vi "Handle Command.vi"(8 "error in (no error)":errorcluster, 9 "Data":variant, 10 "Command":string, 11 "Inst.SPC in":refnum<class "Inst.SPC.lvclass">) -> (0 "error out":errorcluster, 1 "Processed Data":variant, 2 "Command":string, 3 "Inst.SPC out":refnum<class "Inst.SPC.lvclass">)   [LabVIEW 2019, in "Inst.SPC.lvclass"]
uses:
  Inst.SPC.lvclass
  9aec49fd-fe04-463a-be35-b7075f22e824.vi
  <userlib>/LevyLab/Instrument Framework/Instrument Types/VSource/Instrument.VSource.lvclass
  Typedefs/Inst.SPC.Configuration--Cluster.ctl
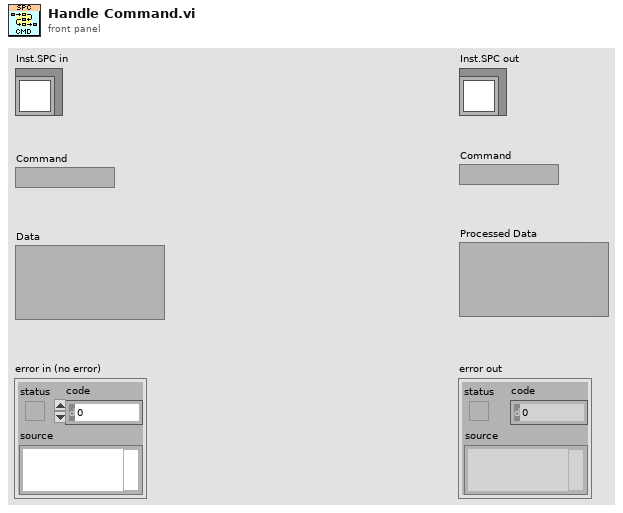
[diagram p1: front panel]
types:
  T1 = typedef "Inst.SPC.lvclass/Inst.SPC.Configuration--Cluster.ctl" = cluster{"DCC_DLL":path, "SPC_DLL":path, "DCC_Serials":string[], "SPC_Serials":string[]}
  T2 = typedef "Inst.SPC.lvclass/Inst.SPC.getAll--Cluster.ctl" = cluster{"DummyData":string}
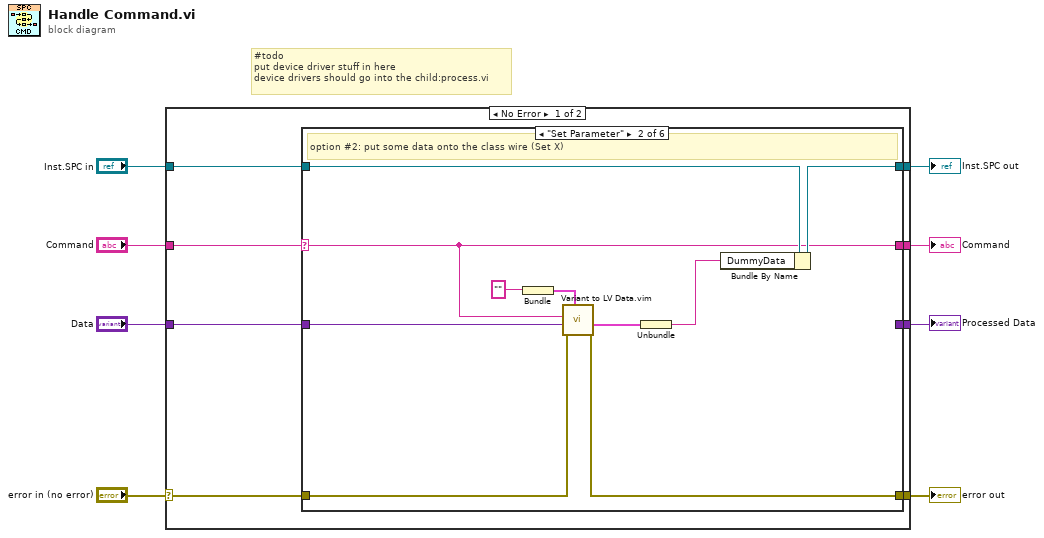
[diagram p0: block diagram]
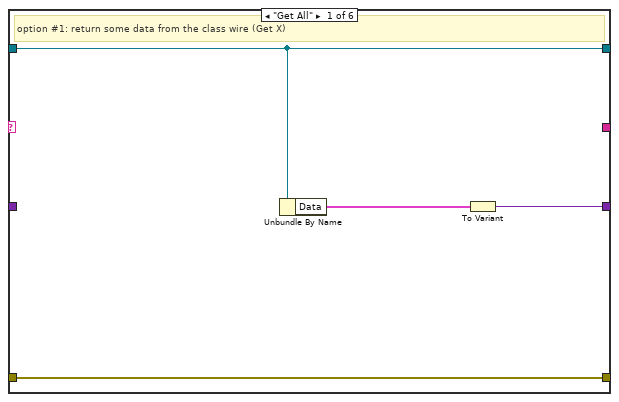
[diagram p2: hidden frame]
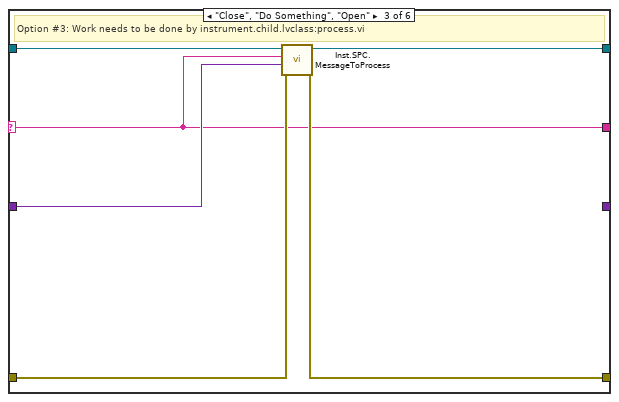
[diagram p3: hidden frame]
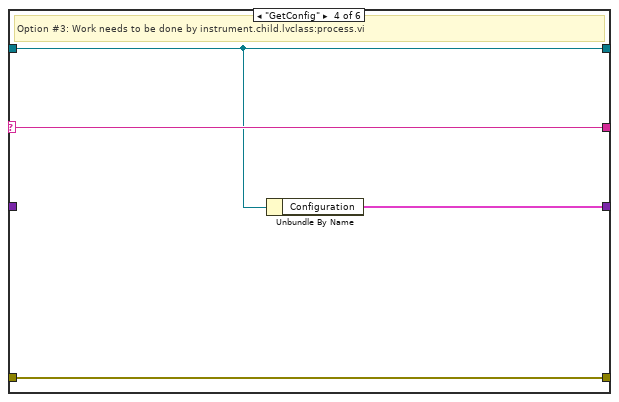
[diagram p4: hidden frame]
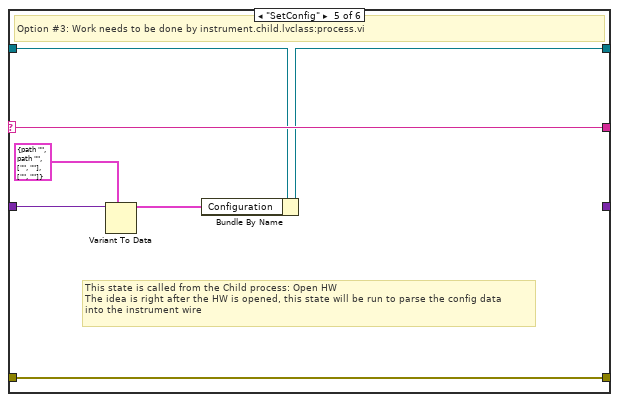
[diagram p5: hidden frame]
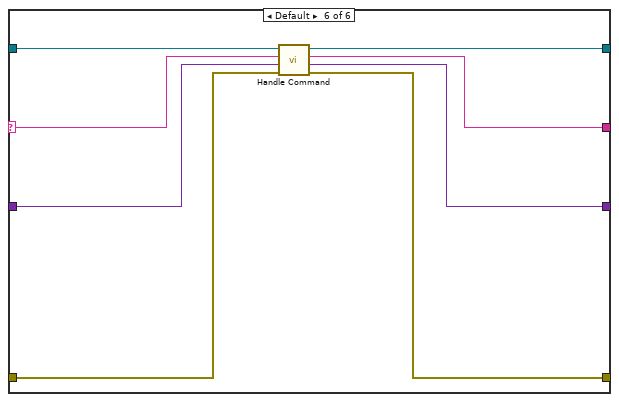
[diagram p6: hidden frame]
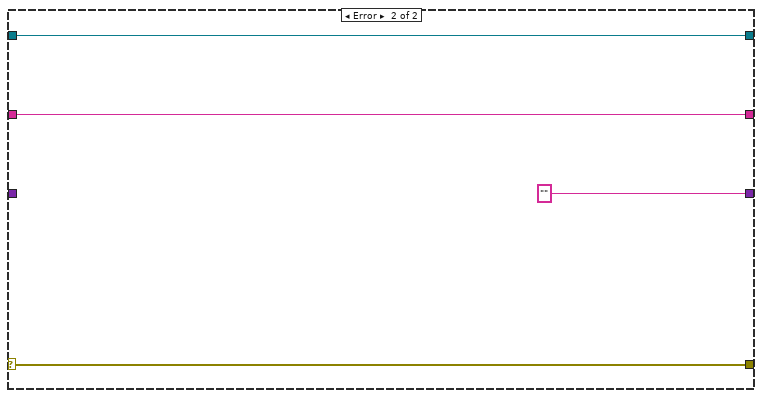
[diagram p7: hidden frame]
diagram:
  # "#todo\nput device driver stuff in here\ndevice drivers should go into the child:process.vi"
  n1 = case shown="No Error" "error in (no error)" {
    selector: "error in (no error)" -> [w10 w59]
    tunnel: [w12 w59] -> w6
    tunnel: [w14 w58] -> w5
    tunnel: "Inst.SPC in" -> [w15 w58]
    tunnel: "Command" -> [w16 w56]
    tunnel: [w13 "" ("String")] -> w3
    tunnel: "Data" -> [w9 _]
    tunnel: [w11 w56] -> w1
    frame No Error {
      n2 = case shown="\"Set Parameter\"" w16 {
        selector: w16 -> [_ w25 w31 w40 w47 w49]
        tunnel: w15 -> [w19 w30 w36 w38 w45 w53]
        tunnel: [w19 w29 w35 w38 w44 w50] -> w14
        tunnel: [w17 _ _ w39 _ w52] -> w13
        tunnel: w10 -> [w18 w28 w34 w37 w46 w54]
        tunnel: w9 -> [_ w26 w32 _ w43 w55]
        tunnel: [w18 w27 w33 w37 w46 w51] -> w12
        tunnel: [_ w25 w31 w40 w47 w48] -> w11
        frame "Get All" {
          # "option #1: return some data from the class wire (Get X)"
          n3 = Unbundle By Name(w19) -> ("Data"=w20:T2)
          n4 = To Variant(anything=w20) -> (Variant=w17:variant)
        }
        frame "Set Parameter" {
          # "option #2: put some data onto the class wire (Set X)"
          n5 = Bundle("") -> (w23:cluster{string})  [unwired: 1 in]
          n6 = call "Variant to LV Data.vim"("type"=w23, "error in (no error)"=w28, "JSON Data in"=w26, "Command"=w25) -> ("error out"=w27:errorcluster, "Data out"=w22:cluster{string})  [unwired: 4 in, 2 out]
          n7 = Unbundle(w22) -> (w21:string)
          n8 = Bundle By Name(cluster=w30, "DummyData"=w21) -> (w29:refnum<class "Inst.SPC.lvclass">)
        }
        frame "Close", "Do Something", "Open" {
          # "Option #3: Work needs to be done by instrument.child.lvclass:process.vi"
          n9 = call "Inst.SPC.MessageToProcess.vi"("error in (no error)"=w34, "Data"=w32, "Command"=w31, "Inst.SPC in"=w36) -> ("error out"=w33:errorcluster, "Inst.SPC out"=w35:refnum<class "Inst.SPC.lvclass">)  [unwired: 6 in]
        }
        frame "GetConfig" {
          # "Option #3: Work needs to be done by instrument.child.lvclass:process.vi"
          n10 = Unbundle By Name(w38) -> ("Configuration"=w39:T1)
        }
        frame "SetConfig" {
          # "This state is called from the Child process: Open HW\nThe idea is right after the HW is opened, this state will be run to parse the config data \ninto the instrument wire"
          # "Option #3: Work needs to be done by instrument.child.lvclass:process.vi"
          n11 = Variant To Data(type=T1 {"DCC_DLL"=path "", "SPC_DLL"=path "", "DCC_Serials"=["", ""], "SPC_Serials"=["", ""]} ("Configuration"), Variant=w43) -> (data=w42:T1)  [unwired: 1 in, 1 out]
          n12 = Bundle By Name(cluster=w45, "Configuration"=w42) -> (w44:refnum<class "Inst.SPC.lvclass">)
        }
        frame Default {
          n13 = call-parent "Handle Command.vi"("error in (no error)"=w54, "Data"=w55, "Command"=w49, "Instrument in"=w53) -> ("error out"=w51:errorcluster, "Processed Data"=w52:variant, "Command"=w48:string, "Instrument out"=w50:refnum<class "Inst.SPC.lvclass">)  [unwired: 4 in]
        }
      }
    }
    frame Error {
    }
  }
  "error out" <- w6
  "Inst.SPC out" <- w5
  "Command" <- w1
  "Processed Data" <- w3
